vi "Tool_Unicode Update Listbox Headers.vi"(6 "Caption":string, 7 "Interpret as Unicode (T)":bool=TRUE, 8 "error in (no error)":errorcluster, 10 "Column Header":string, 11 "Listbox Ref":refnum<vi>) -> (0 "error out":errorcluster, 3 "Listbox Ref":refnum<vi>)   [LabVIEW 2009]
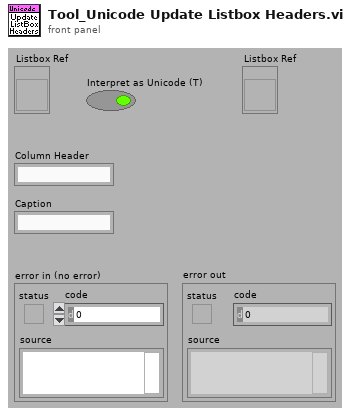
[diagram p1: front panel]
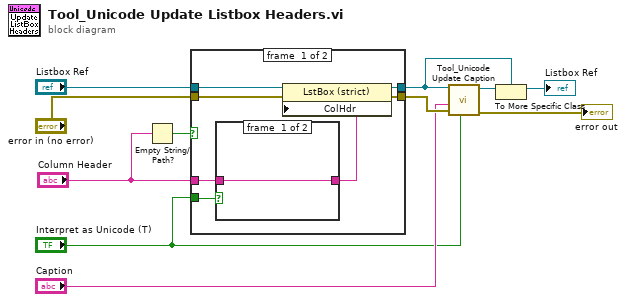
[diagram p0: block diagram]
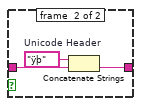
[diagram p2: hidden frame]
diagram:
  n1 = Empty String/Path?(string/path="Column Header") -> (empty?=w11:bool)
  n2 = case shown="False" w11 {
    tunnel: "Column Header" -> [w18 _]
    tunnel: [w17 w24] -> w10
    tunnel: "error in (no error)" -> [w16 w24]
    tunnel: "Listbox Ref" -> [w15 w23]
    tunnel: "Interpret as Unicode (T)" -> [w14 _]
    tunnel: [w13 w23] -> w7
    frame #0 {
      n3 = case shown="True" w14 {
        tunnel: w18 -> [w19 w22]
        tunnel: [w19 w21] -> w12
        frame #0 {
        }
        frame #1 {
          w20 = "ÿþ"  # Unicode Header
          n4 = Concatenate Strings(w20, w22) -> (w21:string)
        }
      }
      n5 = property class="LstBox (strict)"(reference=w15, error in=w16, "ColHdr"=w12) -> (reference out=w13:refnum<vi>, error out=w17:errorcluster)
    }
    frame #1 {
    }
  }
  n6 = call "Tool_Unicode Update Caption.vi"("Interpret as Unicode (T)"="Interpret as Unicode (T)", "error in (no error)"=w10, "Caption"="Caption", "Control Reference"=w7) -> ("error out"=→"error out":errorcluster, "Control Reference"=w8:refnum<vi>)  [unwired: 4 in]
  n7 = To More Specific Class(target class=w7, reference=w8) -> (specific class reference=→"Listbox Ref":refnum<vi>)  [unwired: 1 in, 1 out]
